vi "data-types-sample.vi"() -> ()   [LabVIEW 2020]
panel:
  out "Result 2":dbl
  in  "B-Int32 2":i32
  in  "A-Double 2":dbl
  out "Result":dbl
  in  "B-Int32":i32
  in  "A-Double":dbl
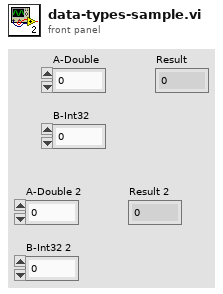
[diagram p1: front panel]
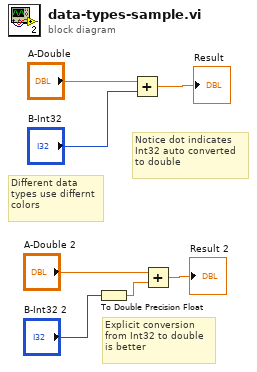
[diagram p0: block diagram]
diagram:
  # "Explicit conversion\nfrom Int32 to double\nis better"
  # "Different data\ntypes use differnt\ncolors"
  # "Notice dot indicates\nInt32 auto converted \nto double"
  n1 = To Double Precision Float(number="B-Int32 2") -> (double precision float=w1:dbl)
  n2 = Add(x="A-Double", y="B-Int32") -> (x+y=→"Result":dbl)
  n3 = Add(x="A-Double 2", y=w1) -> (x+y=→"Result 2":dbl)
